vi "ex_FindNextAvailFileTDM.vi"(8 "error in":errorcluster, 11 "desired file path":path) -> (0 "error out":errorcluster, 3 "next avail file path":path)   [LabVIEW 2017]
panel:
  out "projected 'next avail file path'":path
  out "last 'desired file path'":path
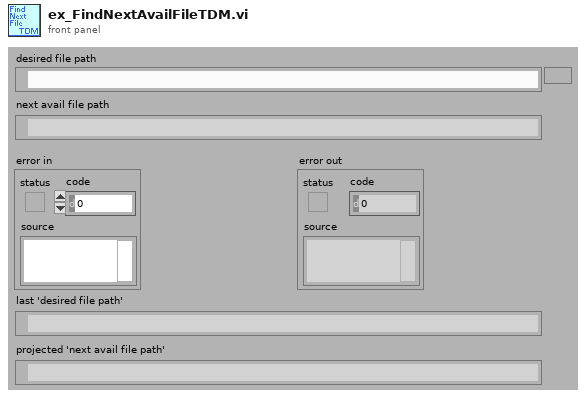
[diagram p1: front panel]
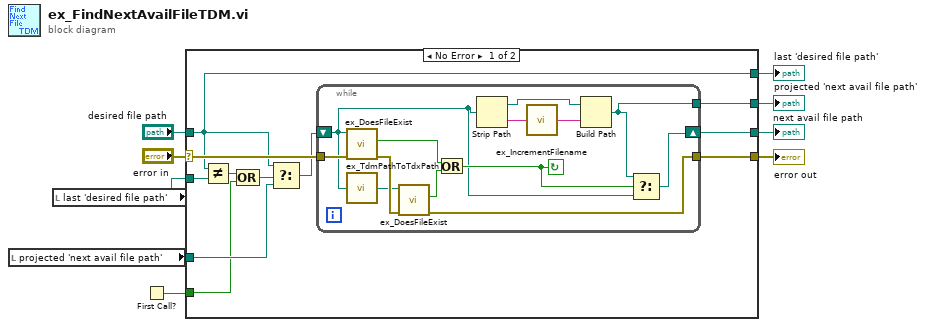
[diagram p0: block diagram]
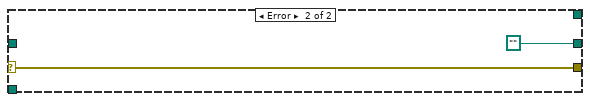
[diagram p2: hidden frame]
diagram:
  n1 = local read "projected 'next avail file path'"() -> (w2:path)
  n2 = local read "last 'desired file path'"() -> (w3:path)
  n3 = First Call?() -> (First Call?: T/F=w1:bool)
  n4 = case shown="No Error" "error in" {
    selector: "error in" -> [w20 w35]
    tunnel: [w19 w35] -> w8
    tunnel: "desired file path" -> [w15 _]
    tunnel: [w18 path ""] -> w6
    tunnel: [w17 _] -> w5
    tunnel: [w15 _] -> w4
    tunnel: w3 -> [w16 _]
    tunnel: w2 -> [w14 _]
    tunnel: w1 -> [w10 _]
    frame No Error {
      n5 = Not Equal?(x=w15, y=w16) -> (x != y?=w11:bool)
      n6 = Compound Arithmetic op=OR(w11, w10) -> (w12:bool)
      n7 = Select(t=w15, s=w12, f=w14) -> (s? t:f=w13:path)
      n8 = while {
        tunnel: w20 -> [w33]
        shift-right: [w32] -> w18
        shift-left: w13 -> [w24]
        tunnel: [w26] -> w19
        tunnel: [w21] -> w17
        stop <- w27 continue-if-true
        n9 = call <vilib>:"ex_DoesFileExist.vi"("error in"=w33, "file path"=w24) -> ("error out"=w31:errorcluster, "file exists"=w29:bool)  [unwired: 4 out]
        n10 = call <vilib>:"ex_TdmPathToTdxPath.vi"("TDM path"=w24) -> ("TDX path"=w30:path)
        n11 = call <vilib>:"ex_DoesFileExist.vi"("error in"=w31, "file path"=w30) -> ("error out"=w26:errorcluster, "file exists"=w28:bool)  [unwired: 4 out]
        n12 = Or(x=w29, y=w28) -> (x .or. y?=w27:bool)
        n13 = Strip Path(path=w24) -> (stripped path=w22:path, name=w25:string)
        n14 = call <vilib>:"ex_IncrementFilename.vi"("name base"=w25) -> ("new name"=w23:string)  [unwired: 4 out]
        n15 = Build Path(base path=w22, name or relative path=w23) -> (appended path=w21:path)
        n16 = Select(t=w21, s=w27, f=w24) -> (s? t:f=w32:path)
      }
    }
    frame Error {
    }
  }
  "error out" <- w8
  "next avail file path" <- w6
  "last 'desired file path'" <- w4
  "projected 'next avail file path'" <- w5
